vi "initCSMs.vi"(8 "error in (no error)":errorcluster, 11 "TestCase in":refnum<class "testcase-CSMChainMode.lvclass">) -> (0 "error out":errorcluster, 3 "TestCase out":refnum<class "testcase-CSMChainMode.lvclass">)   [LabVIEW 2017, in "testcase-CSMChainMode.lvclass"]
uses:
  testcase-CSMChainMode.lvclass
  testcase-CSMChainMode.lvclass/testcase-CSMChainMode.ctl
  CSM/Chain4.vi
  CSM/Chain5.vi
  CSM/Chain6.vi
  <vilib>/addons/_JKI Toolkits/VI Tester/TestCase.llb/TestCase.lvclass
  src/user.lib/_NEVSTOP/Communicable State Machine(CSM)/Communicable State Machine.lvlib
  CSM/CSM-Testcase.lvlib
  C:/Program Files (x86)/National Instruments/LabVIEW 2017/vi.lib/addons/_JKI Toolkits/VI Tester/TestCase.llb/TestCase.lvclass
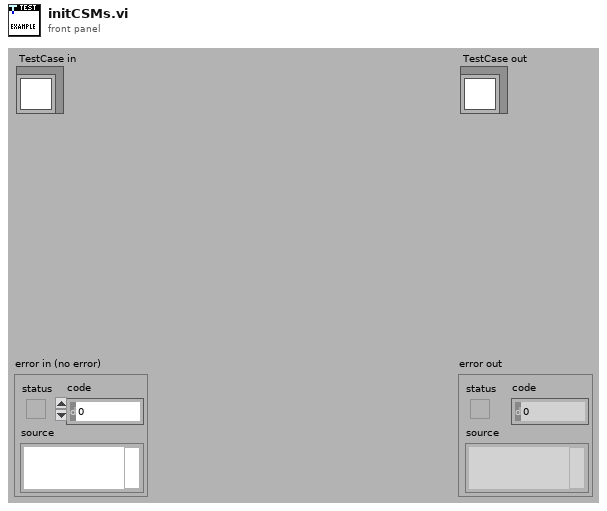
[diagram p1: front panel]
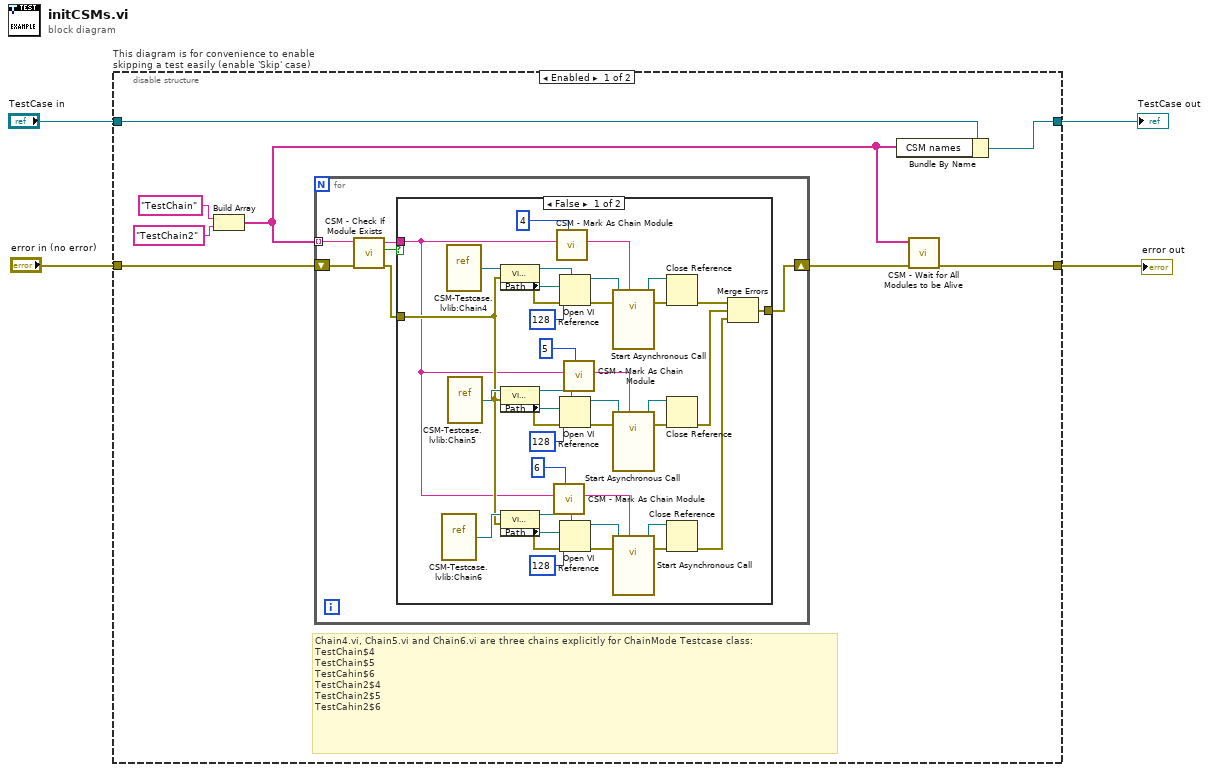
[diagram p0: block diagram]
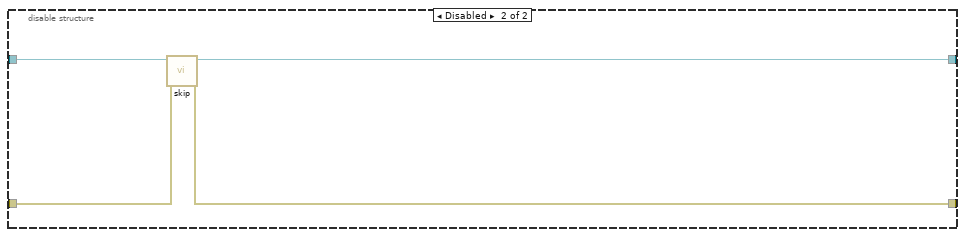
[diagram p3: hidden frame]
diagram:
  n1 = disable-structure "This diagram is for convenience to enable skipping a test easily (enable 'Skip' case)" shown="Enabled" {
    disable-tunnel: "TestCase in" -> [w12 w62]
    disable-tunnel: [w11 w60] -> w1
    disable-tunnel: [w8 w61] -> w3
    disable-tunnel: "error in (no error)" -> [w10 w59]
    frame Enabled {
      # "Chain4.vi, Chain5.vi and Chain6.vi are three chains explicitly for ChainMode Testcase class:\nTestChain$4\nTestChain$5\nTestCahin$6\nTestChain2$4\nTestChain2$5\nTestCahin2$6"
      n2 = Build Array("TestChain" ("CSM Name"), "TestChain2" ("CSM Name")) -> (w5:string[])
      n3 = for {
        tunnel: w5 -> [w15] mode=indexing
        shift-right: [w13] -> w9
        shift-left: w10 -> [w14]
        n4 = call "CSM - Check If Module Exists.vi"("Error In"=w14, "CSM Name"=w15) -> ("error out"=w16:errorcluster, "Exist?"=w18:bool, "CSM Name (Dup)"=w17:string)  [unwired: 7 in]
        n5 = case shown="False" w18 {
          tunnel: [w21 w58] -> w13
          tunnel: w16 -> [w20 w58]
          tunnel: w17 -> [w19 _]
          frame False {
            n6 = vi-ref "CSM-Testcase.lvlib:Chain6.vi"() -> (w39:refnum<vi>)
            n7 = vi-ref "CSM-Testcase.lvlib:Chain4.vi"() -> (w57:refnum<vi>)
            n8 = vi-ref "CSM-Testcase.lvlib:Chain5.vi"() -> (w40:refnum<vi>)
            n9 = property class="VI (strict)"(reference=w57, error in=w20) -> (reference out=w54:refnum<vi>, error out=w52:errorcluster, "Path"=w51:path)
            n10 = property class="VI (strict)"(reference=w40, error in=w20) -> (reference out=w43:refnum<vi>, error out=w45:errorcluster, "Path"=w46:path)
            n11 = property class="VI (strict)"(reference=w39, error in=w20) -> (reference out=w36:refnum<vi>, error out=w34:errorcluster, "Path"=w33:path)
            n12 = call "CSM - Mark As Chain Module.vi"("Order"=6, "CSM Name"=w19) -> ("CSM Name (Marked As Chain)"=w27:string)  [unwired: 8 in]
            n13 = call "CSM - Mark As Chain Module.vi"("Order"=4, "CSM Name"=w19) -> ("CSM Name (Marked As Chain)"=w25:string)  [unwired: 8 in]
            n14 = Open VI Reference(type specifier VI Refnum (for type only)=w54, vi path=w51, options=128, error in (no error)=w52) -> (vi reference=w50:refnum<vi>, error out=w55:errorcluster)  [unwired: 2 in]
            n15 = Open VI Reference(type specifier VI Refnum (for type only)=w43, vi path=w46, options=128, error in (no error)=w45) -> (vi reference=w47:refnum<vi>, error out=w42:errorcluster)  [unwired: 2 in]
            n16 = Open VI Reference(type specifier VI Refnum (for type only)=w36, vi path=w33, options=128, error in (no error)=w34) -> (vi reference=w32:refnum<vi>, error out=w37:errorcluster)  [unwired: 2 in]
            n17 = call "CSM - Mark As Chain Module.vi"("Order"=5, "CSM Name"=w19) -> ("CSM Name (Marked As Chain)"=w26:string)  [unwired: 8 in]
            n18 = call-by-ref "Start Asynchronous Call"(reference=w50, error in=w55, "Name (\"\" to Use UUID)"=w25) -> (reference out=w49:refnum<vi>, error out=w53:errorcluster)  [unwired: 11 in]
            n19 = call-by-ref "Start Asynchronous Call"(reference=w47, error in=w42, "Name (\"\" to Use UUID)"=w26) -> (reference out=w48:refnum<vi>, error out=w44:errorcluster)  [unwired: 11 in]
            n20 = call-by-ref "Start Asynchronous Call"(reference=w32, error in=w37, "Name (\"\" to Use UUID)"=w27) -> (reference out=w31:refnum<vi>, error out=w35:errorcluster)  [unwired: 11 in]
            n21 = Close Reference(reference=w49, error in (no error)=w53) -> (error out=w30:errorcluster)
            n22 = Close Reference(reference=w48, error in (no error)=w44) -> (error out=w29:errorcluster)
            n23 = Close Reference(reference=w31, error in (no error)=w35) -> (error out=w28:errorcluster)
            n24 = Merge Errors(w30, w29, w28) -> (w21:errorcluster)
          }
          frame True {
          }
        }
      }
      n25 = Bundle By Name(cluster=w12, "CSM names"=w5) -> (w11:refnum<class "testcase-CSMChainMode.lvclass">)
      n26 = call "CSM - Wait for All Modules to be Alive.vi"("Error In"=w9, "CSM Names"=w5) -> ("error out"=w8:errorcluster)  [unwired: 7 in, 2 out]
    }
    frame Disabled {
      # "skip test result while test is under development"
      n27 = call <vilib>:"skip.vi"("error in (no error)"=w59, "TestCase in"=w62) -> ("error out"=w61:errorcluster, "TestCase out"=w60:refnum<class "testcase-CSMChainMode.lvclass">)  [unwired: 8 in]
    }
  }
  "error out" <- w3
  "TestCase out" <- w1
